vi "Commands.vi"(7 "Diagnostic Protocol":T2, 10 "Data":dbl[](array[numeric]), 11 "Enum":T1) -> (2 "MetaData":string[](array[string]), 3 "Commands":string[](array[string]))   [LabVIEW 2024, in "Diagnostics Addon Engine.lvlib"]
uses:
  Diagnostics Addon Engine.lvlib
  Addon Shared/Types/Protocol.ctl
  Types/Diagnostics.Command.ctl
  Addon Shared/Types/Command.Memory.ctl
  Addon Shared/Types/Command.IO.ctl
  Addon Shared/Types/Command.ReadDTC.ctl
  Addon Shared/Types/DTC.Descriptor.Override.ctl
  Addon Shared/Types/Command.ReadDTCbyDTCNumber.ctl
  Addon Shared/Types/Command.ClearDTC.ctl
  Addon Shared/Types/Command.ControlDTC.ctl
  Support Libraries/GMLAN/_Types/ReadFailureRecordData_readFailureRecordParameters_failureRecordIdentifier.ctl
  Addon Shared/Types/Command.Communication.ctl
  Addon Shared/Types/Command.PassThru.Channel.ctl
  Addon Shared/Diagnostics Addon Shared.lvlib
  Support Libraries/GMLAN/GMLAN.lvlib
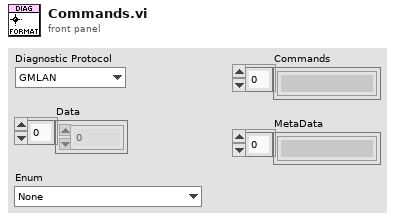
[diagram p1: front panel]
types:
  T1 = typedef "Diagnostics Addon Engine.lvlib/Diagnostics.Command.ctl" = enum8{"None", "Clear Status Channels", "Read DIDs", "Read DID", "Write DID", "Read PIDs", "Read PID", "Write CPID", "Write Memory", "Read Memory", "Input Output Control", "Start Routine", "Request Routine Status", "Stop Routine", "Configure and Start DPIDs", "Stop DPIDs", "Start DTCs", "Read DTCs", "Clear DTCs", "Control DTC", "Read Failure Record Parameters", "Enable Change DTC Count", "Disable Change DTC Count", "Restart Communication", "Close Communication", "Force Tester Present", "Enable Repeating Tester Present", "Disable Repeating Tester Present", "Unlock ECU", "ECU Reset", "Enable Diagnostic Session", "Disable Diagnostic Session", "Disable Normal Communication", "Return To Normal Mode", "Pass Thru Channel Based", "Start Polling", "Stop Polling"}
  T2 = typedef "Diagnostics Addon Shared.lvlib/Protocol.ctl" = enum16{"GMLAN", "KWP-2000", "UDS", "User-Defined"}
  T3 = typedef "Diagnostics Addon Shared.lvlib/Command.Memory.ctl" = cluster{"Address":u64, "Service Type":u32, "Address Length":u8, "Size Length":u8}
  T4 = typedef "Diagnostics Addon Shared.lvlib/Command.IO.ctl" = cluster{"ID":u16, "Mode":u8}
  T5 = typedef "Diagnostics Addon Shared.lvlib/Command.ReadDTC.ctl" = cluster{"Extension":u32, "Mask":u32, "Mode/Status":u32, "Byte Lengths":T6}
  T6 = typedef "Diagnostics Addon Shared.lvlib/DTC.Descriptor.Override.ctl" = cluster{"Override":bool, "DTC":u32, "Status":u32, "Failure":u32}
  T7 = typedef "Diagnostics Addon Shared.lvlib/Command.ReadDTCbyDTCNumber.ctl" = cluster{"DTC":u16, "FailTypeByte":u8}
  T8 = typedef "Diagnostics Addon Shared.lvlib/Command.ClearDTC.ctl" = cluster{"Group of DTC":u32, "Byte Lengths":T6}
  T9 = typedef "Diagnostics Addon Shared.lvlib/Command.ControlDTC.ctl" = cluster{"Group/Type":u32, "Byte Lengths (KWP only)":T6}
  T10 = typedef "GMLAN.lvlib/ReadFailureRecordData_readFailureRecordParameters_failureRecordIdentifier.ctl" = cluster{"failureRecordNumber":u8, "DTC ID":u16, "DTCFailureType":u8}
  T11 = typedef "Diagnostics Addon Shared.lvlib/Command.Communication.ctl" = cluster{"Type":u8, "CommType":u8}
  T12 = typedef "Diagnostics Addon Shared.lvlib/Command.PassThru.Channel.ctl" = cluster{"Service":u64, "Service Length":u8, "Data Length":u32, "Response Required":bool}
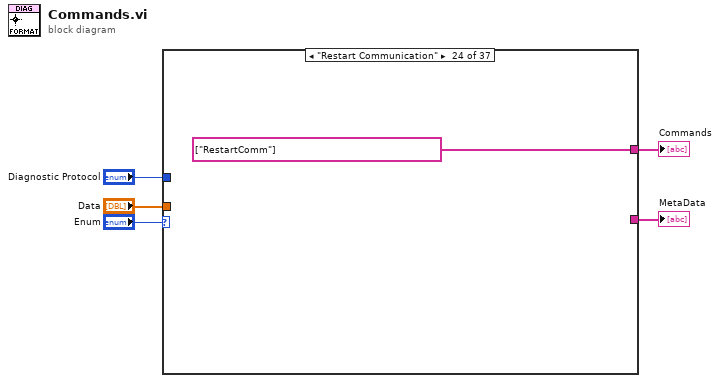
[diagram p0: block diagram]
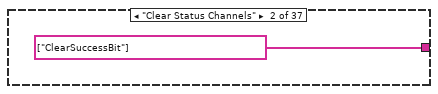
[diagram p3: hidden frame]
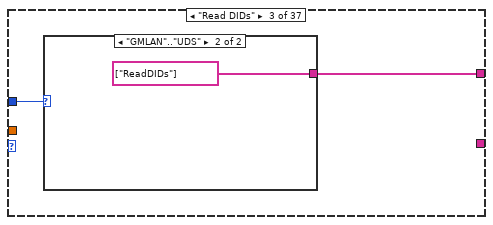
[diagram p4: hidden frame]
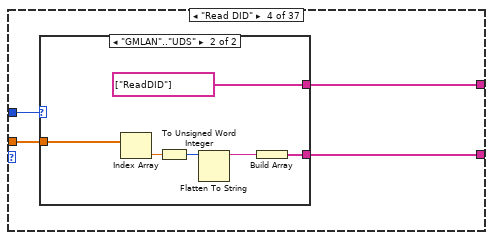
[diagram p6: hidden frame]
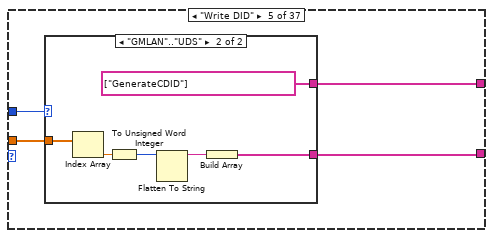
[diagram p8: hidden frame]
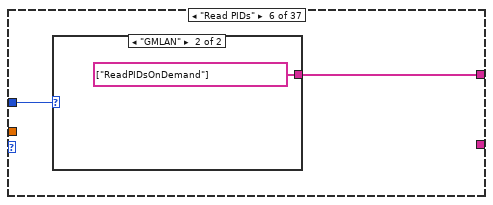
[diagram p10: hidden frame]
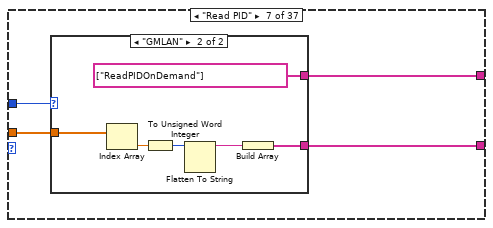
[diagram p12: hidden frame]
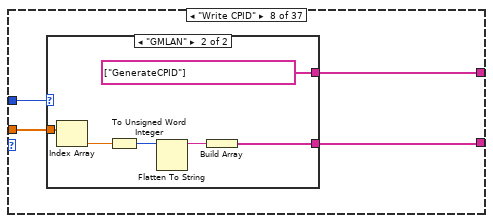
[diagram p14: hidden frame]
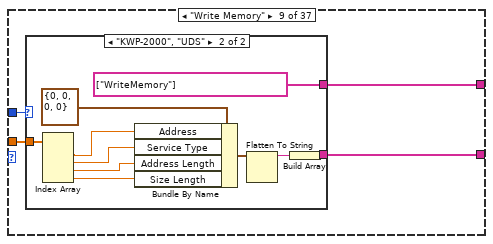
[diagram p16: hidden frame]
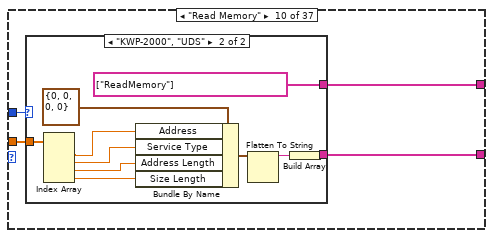
[diagram p18: hidden frame]
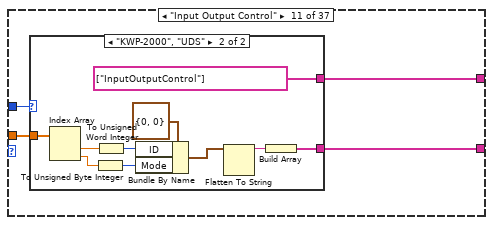
[diagram p20: hidden frame]
diagram:
  n1 = case shown="\"Restart Communication\"" "Enum" {
    tunnel: "Data" -> [_ _ _ w12 w22 _ w35 w45 w54 w68 w82 w96 w106 w116 w128 w138 w149 w159 w188 w214 w243 w260 _ _ _ w279 _ _ w291 w300 w310 _ w323 _ w348 w352 w362]
    tunnel: [_ string[] ["ClearSuccessBit"] w8 w13 w23 w31 w36 w46 w56 w70 w84 w98 w108 w118 w131 w142 w150 w160 w189 w215 w245 w261 w270 string[] ["RestartComm"] string[] ["StopComm"] w280 string[] ["EnableRepeatingTesterPresent"] string[] ["DisableRepeatingTesterPresent"] w293 w301 w311 w319 w324 w336 string[] ["ChannelPassThru"] w353 w363] -> w2
    tunnel: [_ _ _ w11 w21 _ w34 w44 w53 w67 w81 w95 w105 w115 w126 w136 w148 w158 w187 w213 w244 w259 w269 _ _ w278 _ _ w290 w299 w309 _ w322 _ w347 w351 w361] -> w3
    tunnel: "Diagnostic Protocol" -> [_ _ w7 w10 w20 w30 w33 w43 w55 w69 w83 w97 w107 w117 w130 w141 w147 w157 w186 w212 w242 w258 w268 _ _ w277 _ _ w292 w298 w308 w318 w321 w335 _ w350 w360]
    frame "None", Default {
    }
    frame "Clear Status Channels" {
    }
    frame "Read DIDs" {
      n2 = case shown="\"GMLAN\"..\"UDS\"" w7 {
        tunnel: [_ string[] ["ReadDIDs"]] -> w8
        frame "User-Defined" {
        }
        frame "GMLAN".."UDS" {
        }
      }
    }
    frame "Read DID" {
      n3 = case shown="\"GMLAN\"..\"UDS\"" w10 {
        tunnel: [_ string[] ["ReadDID"]] -> w13
        tunnel: w12 -> [_ w15]
        tunnel: [_ w14] -> w11
        frame "User-Defined" {
        }
        frame "GMLAN".."UDS" {
          n4 = Index Array(array=w15) -> (element=w18:dbl)  [unwired: 1 in]
          n5 = To Unsigned Word Integer(number=w18) -> (unsigned 16bit integer=w17:u16)
          n6 = Flatten To String(anything=w17) -> (data string=w16:string)  [unwired: 3 in, 2 out]
          n7 = Build Array(w16) -> (w14:string[])
        }
      }
    }
    frame "Write DID" {
      n8 = case shown="\"GMLAN\"..\"UDS\"" w20 {
        tunnel: [_ string[] ["GenerateCDID"]] -> w23
        tunnel: w22 -> [_ w28]
        tunnel: [_ w27] -> w21
        frame "User-Defined" {
        }
        frame "GMLAN".."UDS" {
          n9 = Index Array(array=w28) -> (element=w26:dbl)  [unwired: 1 in]
          n10 = To Unsigned Word Integer(number=w26) -> (unsigned 16bit integer=w24:u16)
          n11 = Flatten To String(anything=w24) -> (data string=w25:string)  [unwired: 3 in, 2 out]
          n12 = Build Array(w25) -> (w27:string[])
        }
      }
    }
    frame "Read PIDs" {
      n13 = case shown="\"GMLAN\"" w30 {
        tunnel: [_ string[] ["ReadPIDsOnDemand"]] -> w31
        frame Default {
        }
        frame "GMLAN" {
        }
      }
    }
    frame "Read PID" {
      n14 = case shown="\"GMLAN\"" w33 {
        tunnel: [_ string[] ["ReadPIDOnDemand"]] -> w36
        tunnel: w35 -> [_ w38]
        tunnel: [_ w37] -> w34
        frame Default {
        }
        frame "GMLAN" {
          n15 = Index Array(array=w38) -> (element=w41:dbl)  [unwired: 1 in]
          n16 = To Unsigned Word Integer(number=w41) -> (unsigned 16bit integer=w40:u16)
          n17 = Flatten To String(anything=w40) -> (data string=w39:string)  [unwired: 3 in, 2 out]
          n18 = Build Array(w39) -> (w37:string[])
        }
      }
    }
    frame "Write CPID" {
      n19 = case shown="\"GMLAN\"" w43 {
        tunnel: [_ string[] ["GenerateCPID"]] -> w46
        tunnel: w45 -> [_ w51]
        tunnel: [_ w50] -> w44
        frame Default {
        }
        frame "GMLAN" {
          n20 = Index Array(array=w51) -> (element=w49:dbl)  [unwired: 1 in]
          n21 = To Unsigned Word Integer(number=w49) -> (unsigned 16bit integer=w47:u16)
          n22 = Flatten To String(anything=w47) -> (data string=w48:string)  [unwired: 3 in, 2 out]
          n23 = Build Array(w48) -> (w50:string[])
        }
      }
    }
    frame "Write Memory" {
      n24 = case shown="\"KWP-2000\", \"UDS\"" w55 {
        tunnel: [_ string[] ["WriteMemory"]] -> w56
        tunnel: w54 -> [_ w58]
        tunnel: [_ w65] -> w53
        frame "GMLAN", "User-Defined" {
        }
        frame "KWP-2000", "UDS" {
          n25 = Index Array(array=w58) -> (element #1=w62:dbl, element #2=w63:dbl, element #3=w61:dbl, element #4=w60:dbl)  [unwired: 4 in]
          n26 = Bundle By Name(cluster=T3 {"Address"=0, "Service Type"=0, "Address Length"=0, "Size Length"=0}, "Address"=w62, "Service Type"=w63, "Address Length"=w61, "Size Length"=w60) -> (w64:T3)
          n27 = Flatten To String(anything=w64) -> (data string=w59:string)  [unwired: 3 in, 2 out]
          n28 = Build Array(w59) -> (w65:string[])
        }
      }
    }
    frame "Read Memory" {
      n29 = case shown="\"KWP-2000\", \"UDS\"" w69 {
        tunnel: [_ string[] ["ReadMemory"]] -> w70
        tunnel: w68 -> [_ w79]
        tunnel: [_ w77] -> w67
        frame "GMLAN", "User-Defined" {
        }
        frame "KWP-2000", "UDS" {
          n30 = Index Array(array=w79) -> (element #1=w73:dbl, element #2=w74:dbl, element #3=w72:dbl, element #4=w71:dbl)  [unwired: 4 in]
          n31 = Bundle By Name(cluster=T3 {"Address"=0, "Service Type"=0, "Address Length"=0, "Size Length"=0}, "Address"=w73, "Service Type"=w74, "Address Length"=w72, "Size Length"=w71) -> (w75:T3)
          n32 = Flatten To String(anything=w75) -> (data string=w78:string)  [unwired: 3 in, 2 out]
          n33 = Build Array(w78) -> (w77:string[])
        }
      }
    }
    frame "Input Output Control" {
      n34 = case shown="\"KWP-2000\", \"UDS\"" w83 {
        tunnel: [_ string[] ["InputOutputControl"]] -> w84
        tunnel: w82 -> [_ w92]
        tunnel: [_ w85] -> w81
        frame "GMLAN", "User-Defined" {
        }
        frame "KWP-2000", "UDS" {
          n35 = Index Array(array=w92) -> (element #1=w90:dbl, element #2=w91:dbl)  [unwired: 2 in]
          n36 = To Unsigned Byte Integer(number=w91) -> (unsigned 8bit integer=w87:u8)
          n37 = To Unsigned Word Integer(number=w90) -> (unsigned 16bit integer=w88:u16)
          n38 = Bundle By Name(cluster=T4 {"ID"=0, "Mode"=0}, "ID"=w88, "Mode"=w87) -> (w86:T4)
          n39 = Flatten To String(anything=w86) -> (data string=w93:string)  [unwired: 3 in, 2 out]
          n40 = Build Array(w93) -> (w85:string[])
        }
      }
    }
    frame "Start Routine" {
      n41 = case shown="\"KWP-2000\", \"UDS\"" w97 {
        tunnel: [_ string[] ["StartRoutine"]] -> w98
        tunnel: w96 -> [_ w103]
        tunnel: [_ w99] -> w95
        frame "GMLAN", "User-Defined" {
        }
        frame "KWP-2000", "UDS" {
          n42 = Index Array(array=w103) -> (element=w102:dbl)  [unwired: 1 in]
          n43 = To Unsigned Word Integer(number=w102) -> (unsigned 16bit integer=w100:u16)
          n44 = Flatten To String(anything=w100) -> (data string=w101:string)  [unwired: 3 in, 2 out]
          n45 = Build Array(w101) -> (w99:string[])
        }
      }
    }
    frame "Request Routine Status" {
      n46 = case shown="\"KWP-2000\", \"UDS\"" w107 {
        tunnel: [_ string[] ["RequestRoutineStatus"]] -> w108
        tunnel: w106 -> [_ w110]
        tunnel: [_ w109] -> w105
        frame "GMLAN", "User-Defined" {
        }
        frame "KWP-2000", "UDS" {
          n47 = Index Array(array=w110) -> (element=w113:dbl)  [unwired: 1 in]
          n48 = To Unsigned Word Integer(number=w113) -> (unsigned 16bit integer=w111:u16)
          n49 = Flatten To String(anything=w111) -> (data string=w112:string)  [unwired: 3 in, 2 out]
          n50 = Build Array(w112) -> (w109:string[])
        }
      }
    }
    frame "Stop Routine" {
      n51 = case shown="\"KWP-2000\", \"UDS\"" w117 {
        tunnel: [_ string[] ["StopRoutine"]] -> w118
        tunnel: w116 -> [_ w120]
        tunnel: [_ w119] -> w115
        frame "GMLAN", "User-Defined" {
        }
        frame "KWP-2000", "UDS" {
          n52 = Index Array(array=w120) -> (element=w123:dbl)  [unwired: 1 in]
          n53 = To Unsigned Word Integer(number=w123) -> (unsigned 16bit integer=w121:u16)
          n54 = Flatten To String(anything=w121) -> (data string=w122:string)  [unwired: 3 in, 2 out]
          n55 = Build Array(w122) -> (w119:string[])
        }
      }
    }
    frame "Configure and Start DPIDs" {
      n56 = Index Array(array=w128) -> (element=w129:dbl)  [unwired: 1 in]
      n57 = To Unsigned Byte Integer(number=w129) -> (unsigned 8bit integer=w125:u8)
      n58 = Flatten To String(anything=w125) -> (data string=w127:string)  [unwired: 3 in, 2 out]
      n59 = case shown="\"GMLAN\"" w130 {
        tunnel: [_ w133] -> w131
        tunnel: w125 -> [_ w132]
        frame Default {
        }
        frame "GMLAN" {
          n60 = case shown="0" w132 {
            tunnel: [string[] ["EnableDPID"] string[] ["ConfigurePIDs", "StartPIDs"]] -> w133
            frame Default {
            }
            frame 0 {
            }
          }
        }
      }
      n61 = Build Array(w127, w127) -> (w126:string[])
    }
    frame "Stop DPIDs" {
      n62 = Index Array(array=w138) -> (element=w140:dbl)  [unwired: 1 in]
      n63 = To Unsigned Byte Integer(number=w140) -> (unsigned 8bit integer=w137:u8)
      n64 = Flatten To String(anything=w137) -> (data string=w139:string)  [unwired: 3 in, 2 out]
      n65 = Build Array(w139) -> (w136:string[])
      n66 = case shown="\"GMLAN\"" w141 {
        tunnel: [_ w144] -> w142
        tunnel: w137 -> [_ w143]
        frame Default {
        }
        frame "GMLAN" {
          n67 = case shown="Default" w143 {
            tunnel: [string[] ["DisableDPID"] string[] ["StopPIDs"]] -> w144
            frame Default {
            }
            frame 0 {
            }
          }
        }
      }
    }
    frame "Start DTCs" {
      n68 = case shown="\"GMLAN\"" w147 {
        tunnel: [string[] ["StartDTCs"] _] -> w150
        tunnel: w149 -> [w155 _]
        tunnel: [w151 _] -> w148
        frame "GMLAN" {
          n69 = Index Array(array=w155) -> (element=w154:dbl)  [unwired: 1 in]
          n70 = To Unsigned Byte Integer(number=w154) -> (unsigned 8bit integer=w153:u8)
          n71 = Flatten To String(anything=w153) -> (data string=w152:string)  [unwired: 3 in, 2 out]
          n72 = Build Array(w152) -> (w151:string[])
        }
        frame Default {
        }
      }
    }
    frame "Read DTCs" {
      n73 = case shown="\"KWP-2000\", \"UDS\"" w157 {
        tunnel: [string[] ["ReadDTCs"] _ string[] ["ReadDTCByDTCNumber"]] -> w160
        tunnel: w159 -> [w173 _ w182]
        tunnel: [w171 _ w181] -> w158
        frame "KWP-2000", "UDS" {
          n74 = To Unsigned Long Integer(number=w173) -> (unsigned 32bit integer=w175:u32[])
          n75 = Index Array(array=w175) -> (element #1=w167:u32, element #2=w168:u32, element #3=w169:u32, element #4=w163:u32, element #5=w162:u32, element #6=w161:u32)  [unwired: 6 in]
          n76 = Compound Arithmetic op=ADD(w163, w162, w161) -> (w165:u32)
          n77 = Not Equal To 0?(x=w165) -> (x != 0?=w164:bool)
          n78 = Bundle By Name(cluster=T5 {"Extension"=0, "Mask"=0, "Mode/Status"=0, "Byte Lengths"={"Override"=FALSE, "DTC"=0, "Status"=0, "Failure"=0}}, "Extension"=w167, "Mask"=w168, "Mode/Status"=w169, "Byte Lengths.Override"=w164, "Byte Lengths.DTC"=w163, "Byte Lengths.Status"=w162, "Byte Lengths.Failure"=w161) -> (w166:T5)
          n79 = Flatten To String(anything=w166) -> (data string=w174:string)  [unwired: 3 in, 2 out]
          n80 = Build Array(w174) -> (w171:string[])
        }
        frame "User-Defined" {
        }
        frame "GMLAN" {
          n81 = Index Array(array=w182) -> (element #1=w184:dbl, element #2=w180:dbl)  [unwired: 2 in]
          n82 = To Unsigned Word Integer(number=w184) -> (unsigned 16bit integer=w177:u16)
          n83 = To Unsigned Byte Integer(number=w180) -> (unsigned 8bit integer=w179:u8)
          n84 = Bundle By Name(cluster=T7 {"DTC"=0, "FailTypeByte"=0}, "DTC"=w177, "FailTypeByte"=w179) -> (w176:T7)
          n85 = Flatten To String(anything=w176) -> (data string=w183:string)  [unwired: 3 in, 2 out]
          n86 = Build Array(w183) -> (w181:string[])
        }
      }
    }
    frame "Clear DTCs" {
      n87 = case shown="\"KWP-2000\", \"UDS\"" w186 {
        tunnel: [_ string[] ["ClearDTCs"] string[] ["ClearDTCs"]] -> w189
        tunnel: w188 -> [_ w202 w207]
        tunnel: [_ w201 w206] -> w187
        frame "User-Defined" {
        }
        frame "KWP-2000", "UDS" {
          n88 = Index Array(array=w202) -> (element #1=w204:dbl, element #2=w196:dbl, element #3=w195:dbl, element #4=w194:dbl)  [unwired: 4 in]
          n89 = To Unsigned Long Integer(number=w204) -> (unsigned 32bit integer=w199:u32)
          n90 = To Unsigned Long Integer(number=w196) -> (unsigned 32bit integer=w190:u32)
          n91 = To Unsigned Long Integer(number=w195) -> (unsigned 32bit integer=w191:u32)
          n92 = To Unsigned Long Integer(number=w194) -> (unsigned 32bit integer=w192:u32)
          n93 = Compound Arithmetic op=ADD(w190, w191, w192) -> (w197:u32)
          n94 = Not Equal To 0?(x=w197) -> (x != 0?=w193:bool)
          n95 = Bundle By Name(cluster=T8 {"Group of DTC"=16777215, "Byte Lengths"={"Override"=FALSE, "DTC"=0, "Status"=0, "Failure"=0}} ("Clear DTC Settings"), "Group of DTC"=w199, "Byte Lengths.Override"=w193, "Byte Lengths.DTC"=w190, "Byte Lengths.Status"=w191, "Byte Lengths.Failure"=w192) -> (w198:T8)
          n96 = Flatten To String(anything=w198) -> (data string=w203:string)  [unwired: 3 in, 2 out]
          n97 = Build Array(w203) -> (w201:string[])
        }
        frame "GMLAN" {
          n98 = Index Array(array=w207) -> (element=w210:dbl)  [unwired: 1 in]
          n99 = To Unsigned Long Integer(number=w210) -> (unsigned 32bit integer=w209:u32)
          n100 = Flatten To String(anything=w209) -> (data string=w208:string)  [unwired: 3 in, 2 out]
          n101 = Build Array(w208) -> (w206:string[])
        }
      }
    }
    frame "Control DTC" {
      n102 = case shown="\"UDS\"" w212 {
        tunnel: [_ string[] ["ControlDTC"] string[] ["ControlDTC"]] -> w215
        tunnel: w214 -> [_ w228 w238]
        tunnel: [_ w227 w237] -> w213
        frame "GMLAN", "User-Defined" {
        }
        frame "KWP-2000" {
          n103 = Index Array(array=w228) -> (element #1=w230:dbl, element #2=w226:dbl, element #3=w225:dbl, element #4=w224:dbl)  [unwired: 4 in]
          n104 = To Unsigned Long Integer(number=w230) -> (unsigned 32bit integer=w221:u32)
          n105 = To Unsigned Long Integer(number=w226) -> (unsigned 32bit integer=w219:u32)
          n106 = To Unsigned Long Integer(number=w225) -> (unsigned 32bit integer=w218:u32)
          n107 = To Unsigned Long Integer(number=w224) -> (unsigned 32bit integer=w217:u32)
          n108 = Compound Arithmetic op=ADD(w219, w218, w217) -> (w223:u32)
          n109 = Not Equal To 0?(x=w223) -> (x != 0?=w220:bool)
          n110 = Bundle By Name(cluster=T9 {"Group/Type"=16777215, "Byte Lengths (KWP only)"={"Override"=FALSE, "DTC"=0, "Status"=0, "Failure"=0}} ("Clear DTC Settings"), "Group/Type"=w221, "Byte Lengths (KWP only).Override"=w220, "Byte Lengths (KWP only).DTC"=w219, "Byte Lengths (KWP only).Status"=w218, "Byte Lengths (KWP only).Failure"=w217) -> (w216:T9)
          n111 = Flatten To String(anything=w216) -> (data string=w229:string)  [unwired: 3 in, 2 out]
          n112 = Build Array(w229) -> (w227:string[])
        }
        frame "UDS" {
          w232 = u32 0 ("Byte Lengths.DTC")
          n113 = Index Array(array=w238) -> (element=w240:dbl)  [unwired: 1 in]
          n114 = To Unsigned Long Integer(number=w240) -> (unsigned 32bit integer=w235:u32)
          n115 = Bundle By Name(cluster=T9 {"Group/Type"=16777215, "Byte Lengths (KWP only)"={"Override"=FALSE, "DTC"=0, "Status"=0, "Failure"=0}} ("Clear DTC Settings"), "Group/Type"=w235, "Byte Lengths (KWP only).Override"=FALSE ("Byte Lengths.Override"), "Byte Lengths (KWP only).DTC"=w232, "Byte Lengths (KWP only).Status"=w232, "Byte Lengths (KWP only).Failure"=w232) -> (w234:T9)
          n116 = Flatten To String(anything=w234) -> (data string=w239:string)  [unwired: 3 in, 2 out]
          n117 = Build Array(w239) -> (w237:string[])
        }
      }
    }
    frame "Read Failure Record Parameters" {
      n118 = case shown="\"GMLAN\"" w242 {
        tunnel: [_ string[] ["ReadFailureRecordParameters"]] -> w245
        tunnel: [_ w251] -> w244
        tunnel: w243 -> [_ w250]
        frame Default {
        }
        frame "GMLAN" {
          n119 = Index Array(array=w250) -> (element #1=w256:dbl, element #2=w254:dbl, element #3=w246:dbl)  [unwired: 3 in]
          n120 = To Unsigned Word Integer(number=w256) -> (unsigned 16bit integer=w253:u16)
          n121 = To Unsigned Byte Integer(number=w254) -> (unsigned 8bit integer=w248:u8)
          n122 = To Unsigned Byte Integer(number=w246) -> (unsigned 8bit integer=w247:u8)
          n123 = Bundle By Name(cluster=T10 {"failureRecordNumber"=0, "DTC ID"=0, "DTCFailureType"=0} ("failureRecordIdentifier"), "DTC ID"=w253, "DTCFailureType"=w248, "failureRecordNumber"=w247) -> (w252:T10)
          n124 = Flatten To String(anything=w252) -> (data string=w255:string)  [unwired: 3 in, 2 out]
          n125 = Build Array(w255) -> (w251:string[])
        }
      }
    }
    frame "Enable Change DTC Count" {
      n126 = case shown="\"GMLAN\"" w258 {
        tunnel: [_ string[] ["EnableChangeDTCCount"]] -> w261
        tunnel: w260 -> [_ w266]
        tunnel: [_ w262] -> w259
        frame Default {
        }
        frame "GMLAN" {
          n127 = Index Array(array=w266) -> (element=w265:dbl)  [unwired: 1 in]
          n128 = To Unsigned Byte Integer(number=w265) -> (unsigned 8bit integer=w264:u8)
          n129 = Flatten To String(anything=w264) -> (data string=w263:string)  [unwired: 3 in, 2 out]
          n130 = Build Array(w263) -> (w262:string[])
        }
      }
    }
    frame "Disable Change DTC Count" {
      n131 = case shown="\"GMLAN\"" w268 {
        tunnel: [_ string[] ["DisableChangeDTCCount"]] -> w270
        tunnel: [_ w272] -> w269
        frame Default {
        }
        frame "GMLAN" {
          n132 = Flatten To String(anything=u8 0 ("number")) -> (data string=w273:string)  [unwired: 3 in, 2 out]
          n133 = Build Array(w273) -> (w272:string[])
        }
      }
    }
    frame "Restart Communication" {
    }
    frame "Close Communication" {
    }
    frame "Force Tester Present" {
      n134 = case shown="\"GMLAN\"..\"UDS\"" w277 {
        tunnel: [_ string[] ["ForceTesterPresent"]] -> w280
        tunnel: w279 -> [_ w286]
        tunnel: [_ w285] -> w278
        frame "User-Defined" {
        }
        frame "GMLAN".."UDS" {
          n135 = Index Array(array=w286) -> (element=w284:dbl)  [unwired: 1 in]
          n136 = To Unsigned Byte Integer(number=w284) -> (unsigned 8bit integer=w281:u8)
          n137 = Number To Boolean Array(number=w281) -> (Boolean array=w282:bool[])
          n138 = Flatten To String(anything=w282) -> (data string=w283:string)  [unwired: 3 in, 2 out]
          n139 = Build Array(w283) -> (w285:string[])
        }
      }
    }
    frame "Enable Repeating Tester Present" {
    }
    frame "Disable Repeating Tester Present" {
    }
    frame "Unlock ECU" {
      n140 = case shown="\"GMLAN\"..\"UDS\"" w292 {
        tunnel: [_ string[] ["UnlockECU"]] -> w293
        tunnel: w291 -> [_ w296]
        tunnel: [_ w295] -> w290
        frame "User-Defined" {
        }
        frame "GMLAN".."UDS" {
          n141 = call "Format ECU Master Key to String.vi"("Data"=w296) -> ("string"=w294:string)  [unwired: 10 in]
          n142 = Build Array(w294) -> (w295:string[])
        }
      }
    }
    frame "ECU Reset" {
      n143 = case shown="\"KWP-2000\", \"UDS\"" w298 {
        tunnel: [_ string[] ["ECUReset"]] -> w301
        tunnel: w300 -> [_ w303]
        tunnel: [_ w302] -> w299
        frame "GMLAN", "User-Defined" {
        }
        frame "KWP-2000", "UDS" {
          n144 = Index Array(array=w303) -> (element=w306:dbl)  [unwired: 1 in]
          n145 = To Unsigned Byte Integer(number=w306) -> (unsigned 8bit integer=w305:u8)
          n146 = Flatten To String(anything=w305) -> (data string=w304:string)  [unwired: 3 in, 2 out]
          n147 = Build Array(w304) -> (w302:string[])
        }
      }
    }
    frame "Enable Diagnostic Session" {
      n148 = case shown="\"GMLAN\"..\"UDS\"" w308 {
        tunnel: [_ string[] ["EnableDiagnosticSession"]] -> w311
        tunnel: w310 -> [_ w313]
        tunnel: [_ w312] -> w309
        frame "User-Defined" {
        }
        frame "GMLAN".."UDS" {
          n149 = Index Array(array=w313) -> (element=w316:dbl)  [unwired: 1 in]
          n150 = To Unsigned Byte Integer(number=w316) -> (unsigned 8bit integer=w315:u8)
          n151 = Flatten To String(anything=w315) -> (data string=w314:string)  [unwired: 3 in, 2 out]
          n152 = Build Array(w314) -> (w312:string[])
        }
      }
    }
    frame "Disable Diagnostic Session" {
      n153 = case shown="\"GMLAN\"..\"UDS\"" w318 {
        tunnel: [_ string[] ["DisableDiagnosticSession"]] -> w319
        frame "User-Defined" {
        }
        frame "GMLAN".."UDS" {
        }
      }
    }
    frame "Disable Normal Communication" {
      n154 = case shown="\"GMLAN\"..\"UDS\"" w321 {
        tunnel: [_ string[] ["DisableNormalCommunication"]] -> w324
        tunnel: w323 -> [_ w326]
        tunnel: [_ w325] -> w322
        frame "User-Defined" {
        }
        frame "GMLAN".."UDS" {
          n155 = Index Array(array=w326) -> (element #1=w331:dbl, element #2=w332:dbl)  [unwired: 2 in]
          n156 = To Unsigned Byte Integer(number=w332) -> (unsigned 8bit integer=w329:u8)
          n157 = To Unsigned Byte Integer(number=w331) -> (unsigned 8bit integer=w330:u8)
          n158 = Bundle By Name(cluster=T11 {"Type"=0, "CommType"=0} ("Cluster"), "Type"=w330, "CommType"=w329) -> (w328:T11)
          n159 = Flatten To String(anything=w328) -> (data string=w333:string)  [unwired: 3 in, 2 out]
          n160 = Build Array(w333) -> (w325:string[])
        }
      }
    }
    frame "Return To Normal Mode" {
      n161 = case shown="\"GMLAN\"..\"UDS\"" w335 {
        tunnel: [_ string[] ["ReturnToNormalMode"]] -> w336
        frame "User-Defined" {
        }
        frame "GMLAN".."UDS" {
        }
      }
    }
    frame "Pass Thru Channel Based" {
      n162 = Index Array(array=w348) -> (element #1=w344:dbl, element #2=w345:dbl, element #3=w343:dbl, element #4=w340:dbl)  [unwired: 4 in]
      n163 = To Unsigned Byte Integer(number=w340) -> (unsigned 8bit integer=w339:u8)
      n164 = Greater Than 0?(x=w339) -> (x > 0?=w338:bool)
      n165 = Bundle By Name(cluster=T12 {"Service"=0, "Service Length"=0, "Data Length"=0, "Response Required"=FALSE}, "Service"=w344, "Service Length"=w345, "Data Length"=w343, "Response Required"=w338) -> (w346:T12)
      n166 = Flatten To String(anything=w346) -> (data string=w342:string)  [unwired: 3 in, 2 out]
      n167 = Build Array(w342) -> (w347:string[])
    }
    frame "Start Polling" {
      n168 = case shown="\"GMLAN\"..\"UDS\"" w350 {
        tunnel: [_ string[] ["StartPolling"]] -> w353
        tunnel: w352 -> [_ w355]
        tunnel: [_ w354] -> w351
        frame "User-Defined" {
        }
        frame "GMLAN".."UDS" {
          n169 = Index Array(array=w355) -> (element=w358:dbl)  [unwired: 1 in]
          n170 = To Unsigned Long Integer(number=w358) -> (unsigned 32bit integer=w357:u32)
          n171 = Flatten To String(anything=w357) -> (data string=w356:string)  [unwired: 3 in, 2 out]
          n172 = Build Array(w356) -> (w354:string[])
        }
      }
    }
    frame "Stop Polling" {
      n173 = case shown="\"GMLAN\"..\"UDS\"" w360 {
        tunnel: [_ string[] ["StopPolling"]] -> w363
        tunnel: w362 -> [_ w365]
        tunnel: [_ w364] -> w361
        frame "User-Defined" {
        }
        frame "GMLAN".."UDS" {
          n174 = Index Array(array=w365) -> (element=w368:dbl)  [unwired: 1 in]
          n175 = To Unsigned Long Integer(number=w368) -> (unsigned 32bit integer=w367:u32)
          n176 = Flatten To String(anything=w367) -> (data string=w366:string)  [unwired: 3 in, 2 out]
          n177 = Build Array(w366) -> (w364:string[])
        }
      }
    }
  }
  "MetaData" <- w3
  "Commands" <- w2
